vi "Process Secret Number.vi"(11 "Starting Secret Number":u64) -> (3 "New Secret Number":u64)   [LabVIEW 2024]
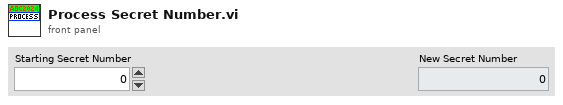
[diagram p1: front panel]
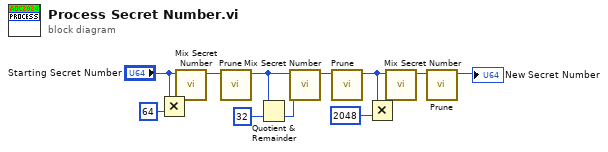
[diagram p0: block diagram]
diagram:
  n1 = Multiply(x="Starting Secret Number", y=u64 64) -> (x*y=w4:u64)
  n2 = call "Mix Secret Number.vi"("Value"=w4, "Current Secret Number"="Starting Secret Number") -> ("New Secret Number"=w6:u64)  [unwired: 9 in]
  n3 = call "Prune.vi"("Secret Number"=w6) -> ("New Secret Number"=w8:u64)  [unwired: 10 in]
  n4 = Quotient & Remainder(x=w8, y=u64 32) -> (floor(x/y)=w1:u64)  [unwired: 1 out]
  n5 = call "Mix Secret Number.vi"("Value"=w1, "Current Secret Number"=w8) -> ("New Secret Number"=w9:u64)  [unwired: 9 in]
  n6 = call "Prune.vi"("Secret Number"=w9) -> ("New Secret Number"=w12:u64)  [unwired: 10 in]
  n7 = Multiply(x=w12, y=u64 2048) -> (x*y=w11:u64)
  n8 = call "Mix Secret Number.vi"("Value"=w11, "Current Secret Number"=w12) -> ("New Secret Number"=w13:u64)  [unwired: 9 in]
  n9 = call "Prune.vi"("Secret Number"=w13) -> ("New Secret Number"=→"New Secret Number":u64)  [unwired: 10 in]
